vi "FTW-Panel-FrontPanel-Hide.vi"(8 "error in":errorcluster, 11 "VI Ref":refnum<vi>) -> (0 "error out":errorcluster, 3 "VI Ref out":refnum<vi>)   [LabVIEW 2015]
panel:
  # "Inputs"
  # "Outputs"
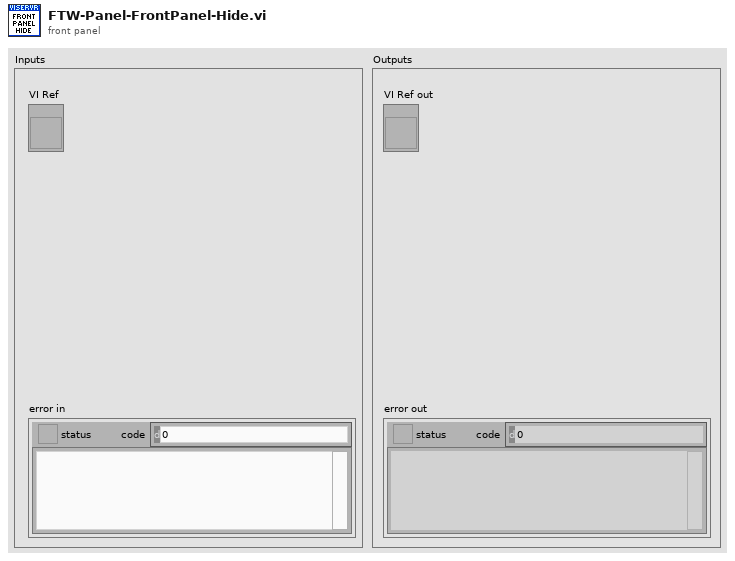
[diagram p1: front panel]
types:
  T1 = enum32{"Invalid", "Standard", "Closed", "Hidden", "Minimized", "Maximized"}
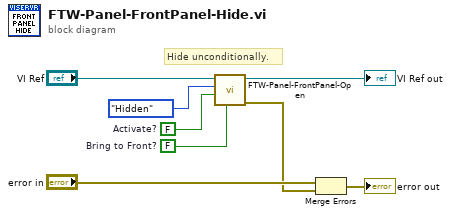
[diagram p0: block diagram]
diagram:
  w1 = FALSE  # Bring to Front?
  w5 = FALSE  # Activate?
  # "Hide unconditionally."
  n1 = call "FTW-Panel-FrontPanel-Open.vi"("Bring to Front?"=w1, "Activate?"=w5, "State"=T1."Hidden", "VI Ref"="VI Ref") -> ("error out"=w2:errorcluster, "VI Ref out"=→"VI Ref out":refnum<vi>)  [unwired: 6 in]
  n2 = Merge Errors("error in", w2) -> (→"error out":errorcluster)
